vi "Bank.vi"() -> ()   [LabVIEW 2015]
doc: "This VI simulates the transactions that occur in a bank and demonstrates race conditions.\n\nRun the VI, and attempt a simultaneous transaction and notice that either the withdrawal or deposit is lost. Try to find and solve the problem."
panel:
  out "Balance":dbl
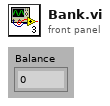
[diagram p1: front panel]
types:
  T1 = typedef "Account Info.ctl" = cluster{"Bank Rendezvous":T2, "Withdrawal Queue":refnum<queue>, "Deposit Queue":refnum<queue>}
  T2 = typedef "Rendezvous RefNum" = refnum<k1>
  T3 = typedef "Semaphore RefNum" = refnum<k1>
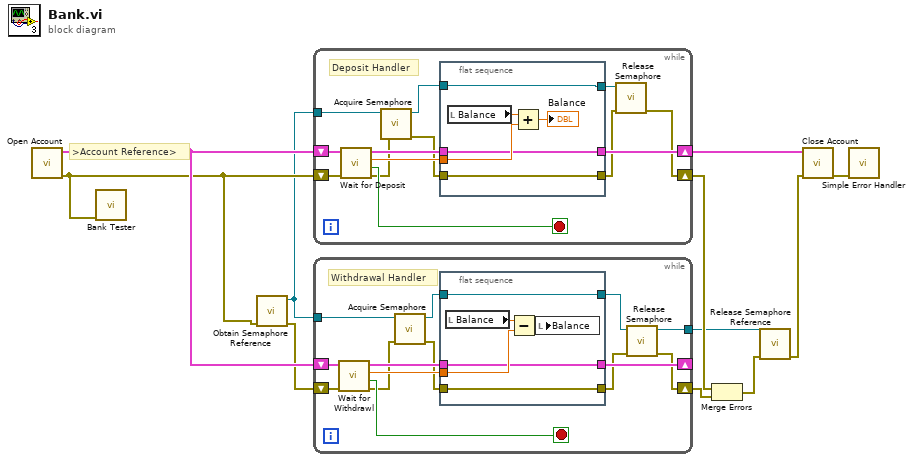
[diagram p0: block diagram]
diagram:
  # ">Account Reference>"
  n1 = call "Open Account.vi"() -> ("error out"=w6:errorcluster, "Account info"=w11:T1)  [unwired: 10 in]
  n2 = call "Bank Tester.vi"("error in (no error)"=w6) -> ()  [unwired: 10 in, 1 out]
  n3 = call <vilib>:"Obtain Semaphore Reference.vi"("error in (no error)"=w6) -> ("error out"=w5:errorcluster, "semaphore"=w2:T3)  [unwired: 4 in, 1 out]
  n4 = while {
    shift-right: [w20] -> w8
    shift-left: w11 -> [w23]
    shift-right: [w15] -> w10
    shift-left: w6 -> [w22]
    tunnel: w2 -> [w16]
    stop <- w19 stop-if-true
    # "Deposit Handler"
    n5 = call "Wait for Deposit.vi"("error in (no error)"=w22, "Account info"=w23) -> ("error out"=w18:errorcluster, "Stop?"=w19:bool, "Deposit Amount"=w24:dbl, "Account info out"=w21:T1)  [unwired: 6 in]
    n6 = call <vilib>:"Acquire Semaphore.vi"("error in (no error)"=w18, "semaphore"=w16) -> ("error out"=w17:errorcluster, "semaphore out"=w12:T3)  [unwired: 3 in, 1 out]
    n7 = flat-sequence {
      tunnel: w24 -> [w30]
      tunnel: [w27] -> w20
      tunnel: w21 -> [w27]
      tunnel: w17 -> [w26]
      tunnel: [w26] -> w14
      tunnel: [w25] -> w13
      tunnel: w12 -> [w25]
      frame #0 {
        n8 = local read "Balance"() -> (w28:dbl)
        n9 = Add(x=w28, y=w30) -> (x+y=→"Balance":dbl)
      }
    }
    n10 = call <vilib>:"Release Semaphore.vi"("error in (no error)"=w14, "semaphore"=w13) -> ("error out"=w15:errorcluster)  [unwired: 4 in, 1 out]
  }
  n11 = while {
    shift-right: [w40] -> _
    shift-left: w11 -> [w43]
    shift-right: [w36] -> w9
    shift-left: w5 -> [w42]
    tunnel: w2 -> [w34]
    tunnel: [w31] -> w1
    stop <- w39 stop-if-true
    # "Withdrawal Handler"
    n12 = call "Wait for Withdrawl.vi"("error in (no error)"=w42, "Account info"=w43) -> ("error out"=w38:errorcluster, "Stop?"=w39:bool, "Withdrawal Amount"=w44:dbl, "Account info out"=w41:T1)  [unwired: 6 in]
    n13 = call <vilib>:"Acquire Semaphore.vi"("error in (no error)"=w38, "semaphore"=w34) -> ("error out"=w37:errorcluster, "semaphore out"=w32:T3)  [unwired: 3 in, 1 out]
    n14 = flat-sequence {
      tunnel: w44 -> [w48]
      tunnel: w41 -> [w47]
      tunnel: w37 -> [w46]
      tunnel: [w47] -> w40
      tunnel: [w46] -> w35
      tunnel: [w45] -> w33
      tunnel: w32 -> [w45]
      frame #0 {
        n15 = local read "Balance"() -> (w49:dbl)
        n16 = Subtract(x=w49, y=w48) -> (x-y=w50:dbl)
        n17 = local write "Balance"(w50) -> ()
      }
    }
    n18 = call <vilib>:"Release Semaphore.vi"("error in (no error)"=w35, "semaphore"=w33) -> ("error out"=w36:errorcluster, "semaphore out"=w31:T3)  [unwired: 4 in]
  }
  n19 = Merge Errors(w10, w9) -> (w4:errorcluster)
  n20 = call <vilib>:"Release Semaphore Reference.vi"("error in (no error)"=w4, "semaphore"=w1) -> ("error out"=w3:errorcluster)  [unwired: 8 in, 1 out]
  n21 = call "Close Account.vi"("error in"=w3, "Account info"=w8) -> ("error out"=w7:errorcluster)  [unwired: 9 in]
  n22 = call <vilib>:"Simple Error Handler.vi"("error in (no error)"=w7) -> ()  [unwired: 4 in, 5 out]
